vi "zlib Uncompress.vi"(8 "error in (no error)":errorcluster, 10 "Uncompressed Size in":u32, 11 "Compressed Data in":string) -> (0 "error out":errorcluster, 2 "Uncompressed Size out":i32, 3 "Uncompressed Data out":string)   [LabVIEW 2018, in "VI-Hacker.lvlib"]
uses:
  VI-Hacker.lvlib
  <vilib>/ErrorRing/Error Ring.xnode
  <vilib>/Utility/error.llb/Error Cluster From Error Code.vi
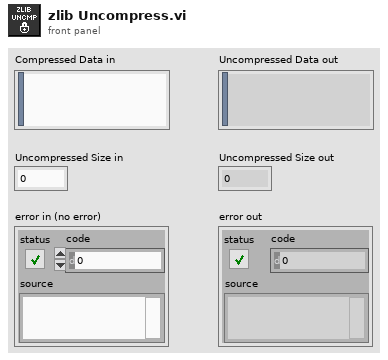
[diagram p1: front panel]
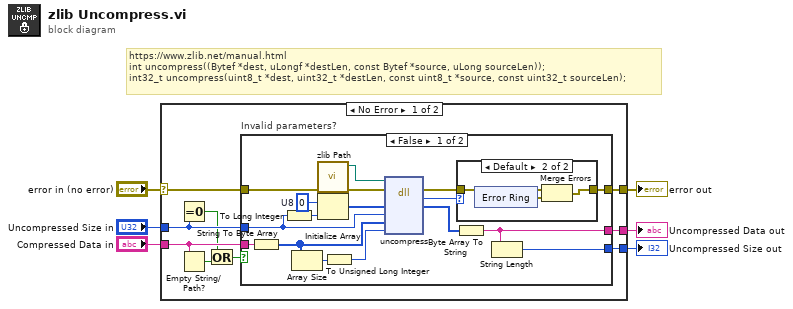
[diagram p0: block diagram]
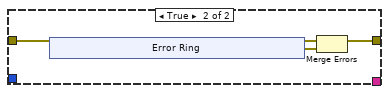
[diagram p3: hidden frame]
diagram:
  # "https://www.zlib.net/manual.html\nint uncompress((Bytef *dest, uLongf *destLen, const Bytef *source, uLong sourceLen));\nint32_t uncompress(uint8_t *dest, uint32_t *destLen, const uint8_t *source, const uint32_t sourceLen);"
  n1 = case shown="No Error" "error in (no error)" {
    selector: "error in (no error)" -> [w15 w49]
    tunnel: "Uncompressed Size in" -> [w12 _]
    tunnel: "Compressed Data in" -> [w11 _]
    tunnel: [w14 w49] -> w3
    tunnel: [w13 _] -> w2
    tunnel: [w7 _] -> w1
    frame No Error {
      n2 = Equal To 0?(x=w12) -> (x = 0?=w9:bool)
      n3 = Empty String/Path?(string/path=w11) -> (empty?=w10:bool)
      n4 = Or(x=w9, y=w10) -> (x .or. y?=w8:bool)
      n5 = case "Invalid parameters?" shown="False" w8 {
        tunnel: w15 -> [w17 w42]
        tunnel: w12 -> [w30 _]
        tunnel: w11 -> [w29 _]
        tunnel: [w22 w41] -> w14
        tunnel: [w20 _] -> w13
        tunnel: [w19 _] -> w7
        frame False {
          w32 = u8 0  # U8
          n6 = String To Byte Array(string=w29) -> (unsigned byte array=w26:u8[])
          n7 = To Long Integer(number=w30) -> (32bit integer=w27:i32)
          n8 = Array Size(array=w26) -> (size(s)=w25:i32)
          n9 = call "zlib Path.vi"("error in (no error)"=w17) -> ("error out"=w18:errorcluster, "zlib.dll Path"=w16:path)  [unwired: 8 in, 1 out]
          n10 = Initialize Array(w32, w27) -> (w31:u8[])
          n11 = To Unsigned Long Integer(number=w25) -> (unsigned 32bit integer=w28:u32)
          n12 = dll-call lib="zlib.dll" fn="uncompress"(path in=w16, error in=w18, "dest"=w31, "destLen"=w30, "source"=w26, "sourceLen"=w28) -> (error out=w23:errorcluster, "return type"=w24:i32, "dest"=w21:u8[])  [unwired: 4 in, 1 out]
          n13 = Byte Array To String(unsigned byte array=w21) -> (string=w20:string)
          n14 = case shown="Default" w24 {
            tunnel: w23 -> [w33 w36]
            tunnel: [w33 w35] -> w22
            frame 0 {
            }
            frame Default {
              n15 = xnode "Error Ring"() -> ("error out"=w34:errorcluster)
              n16 = Merge Errors(w36, w34) -> (w35:errorcluster)
            }
          }
          n17 = String Length(string=w20) -> (length=w19:i32)
        }
        frame True {
          n18 = xnode "Error Ring"() -> ("error out"=w43:errorcluster)
          n19 = Merge Errors(w42, w43) -> (w41:errorcluster)
        }
      }
    }
    frame Error {
    }
  }
  "error out" <- w3
  "Uncompressed Data out" <- w2
  "Uncompressed Size out" <- w1
